vi "读取测试数据.vi"(8 "错误输入（无错误）":errorcluster, 11 "VISA资源名称":refnum<visa-resource-name>) -> (0 "错误输出":errorcluster, 1 "完成":bool, 2 "测试数据":dbl[][](array[numeric]), 3 "VISA资源名称输出":refnum<visa-resource-name>, 5 "read buffer":string)   [LabVIEW 2021]
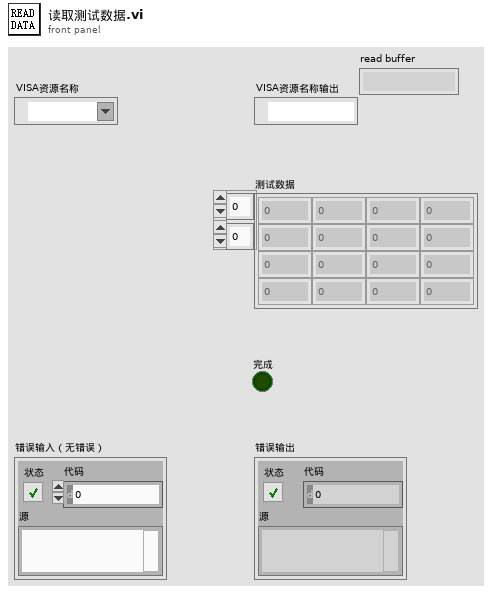
[diagram p1: front panel]
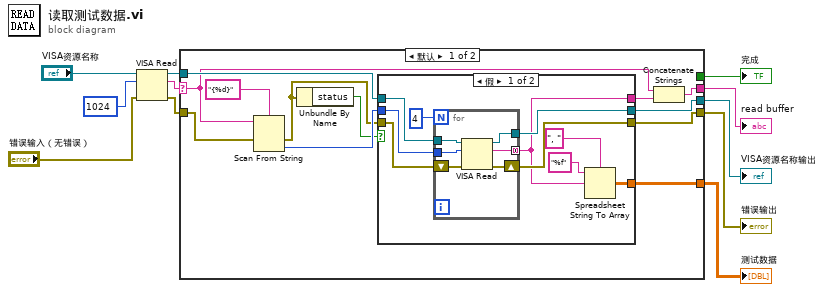
[diagram p0: block diagram]
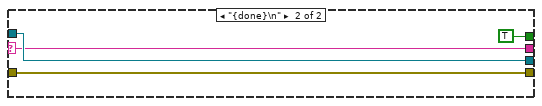
[diagram p3: hidden frame]
diagram:
  n1 = VISA Read(VISA resource name="VISA资源名称", byte count=u32 1024 ("字节总数"), error in (no error)="错误输入（无错误）") -> (VISA resource name out=w6:refnum<visa-resource-name>, read buffer=w9:string, error out=w7:errorcluster)  [unwired: 1 out]
  n2 = case shown="默认" w9 {
    selector: w9 -> [w14 w42]
    tunnel: w7 -> [w21 w45]
    tunnel: [w20 w45] -> w4
    tunnel: [w19 w44] -> w5
    tunnel: [w18 _] -> w2
    tunnel: w6 -> [w17 w44]
    tunnel: [_ TRUE] -> w3
    tunnel: [w12 w42] -> w1
    frame Default {
      n3 = Scan From String(format string="{%d}" ("格式字符串"), input string=w14, error in=w21) -> (error out=w16:errorcluster, output 1=w23:i32)  [unwired: 2 in, 2 out]
      n4 = Unbundle By Name(w16) -> ("status"=w15:bool)
      n5 = case shown="假" w15 {
        tunnel: w23 -> [w25 _]
        tunnel: [w30 w40] -> w20
        tunnel: [w29 w41] -> w19
        tunnel: [w26 _] -> w18
        tunnel: w17 -> [w28 w41]
        tunnel: w16 -> [w27 w40]
        tunnel: [w24 _] -> w13
        frame False {
          n6 = for {
            N: 4 -> [_]
            tunnel: [w37] -> w29
            tunnel: w25 -> [w36]
            tunnel: [w35] -> w24 mode=concatenating
            shift-right: [w38] -> w30
            shift-left: w27 -> [w39]
            tunnel: w28 -> [w34]
            n7 = VISA Read(VISA resource name=w34, byte count=w36, error in (no error)=w39) -> (VISA resource name out=w37:refnum<visa-resource-name>, read buffer=w35:string, error out=w38:errorcluster)  [unwired: 1 out]
          }
          n8 = Spreadsheet String To Array(delimiter (Tab)=", " ("分隔符(Tab)"), format string="%f" ("格式字符串"), spreadsheet string=w24) -> (array=w26:dbl[][])  [unwired: 1 in]
        }
        frame True {
        }
      }
      n9 = Concatenate Strings(w14, w13) -> (w12:string)
    }
    frame "{done}\n" {
    }
  }
  "VISA资源名称输出" <- w5
  "错误输出" <- w4
  "完成" <- w3
  "测试数据" <- w2
  "read buffer" <- w1
